vi "MMI_PEPS_StrDismantle.vi"(1 "LogEvent":refnum<vi>, 2 "VCI_CAN_OBJ_R":T1) -> (0 "MMI_PEPS_CmdCluster":T2 {"任意门开启锁车报警" items=["无请求", "禁止", "启用", "预留"]; "天窗/遮阳帘关闭设置" items=["无请求", "天窗关闭", "遮阳帘关闭", "预留"]; "车窗透气开启设置" items=["无请求", "禁止", "启用", "预留"]; "前雨刮激活后雨刮" items=["无请求", "不激活", "激活", "预留"]; "AVM道路中标定请求" items=["无请求", "开始标定", "预留"]; "自动开关窗设置" items=["无请求", "RKE长按控制", "车钥匙控制", "预留"]; "迎宾灯功能开关" items=["无请求", "禁止", "启用", "预留"]; "钥匙忘车内锁车报警" items=["无请求", "禁止", "启用", "预留"]; "AVAS禁用设置" items=["无请求", "禁止", "启用", "预留"]; "电源非OFF锁车报警" items=["无请求", "禁止", "启用", "预留"]; "外后视镜倒车倾斜" items=["无请求", "禁止所有倾斜", "启用驾驶侧", "启用乘客侧", "启用所有侧"]})   [LabVIEW 2013]
uses:
  Log.ctl
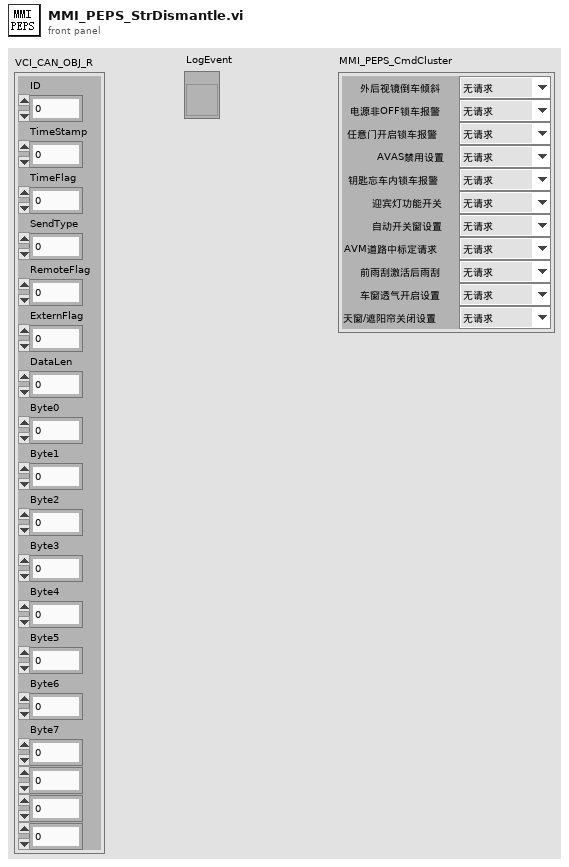
[diagram p1: front panel]
types:
  T1 = cluster{"ID":u32, "TimeStamp":u32, "TimeFlag":u8, "SendType":u8, "RemoteFlag":u8, "ExternFlag":u8, "DataLen":u8, "Byte0":u8, "Byte1":u8, "Byte2":u8, "Byte3":u8, "Byte4":u8, "Byte5":u8, "Byte6":u8, "Byte7":u8, u8, u8, u8}
  T2 = cluster{"外后视镜倒车倾斜":u16, "电源非OFF锁车报警":u16, " 任意门开启锁车报警":u16, "AVAS禁用设置":u16, "钥匙忘车内锁车报警":u16, "迎宾灯功能开关":u16, "自动开关窗设置":u16, "AVM道路中标定请求":u16, "前雨刮激活后雨刮":u16, "车窗透气开启设置":u16, "天窗/遮阳帘关闭设置":u16}
  T3 = typedef "Log.ctl" = cluster{"Event":string, "Value":variant}
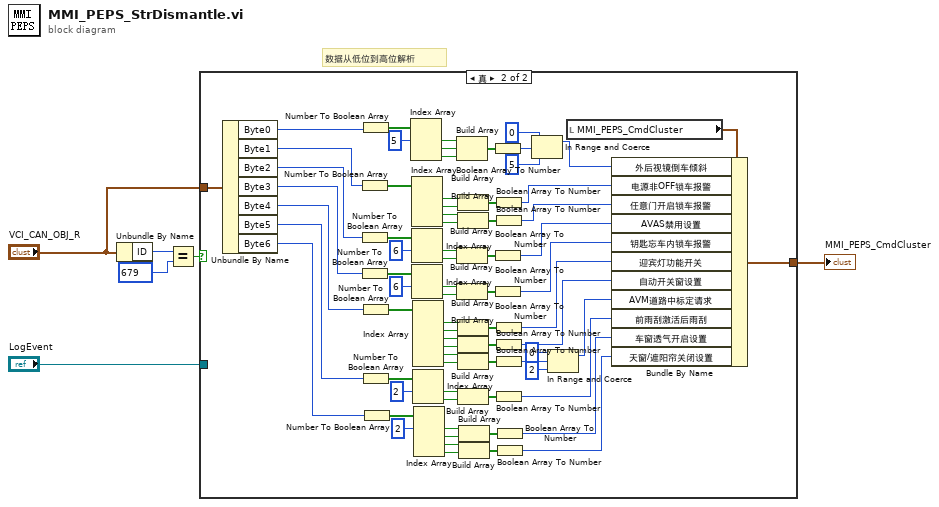
[diagram p0: block diagram]
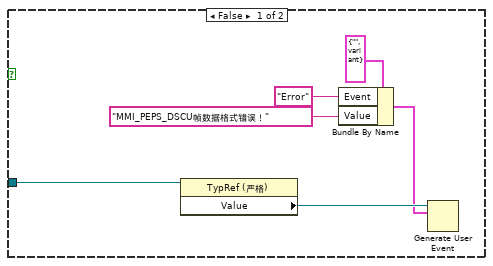
[diagram p2: hidden frame]
diagram:
  # "数据从低位到高位解析"
  n1 = Unbundle By Name("VCI_CAN_OBJ_R") -> ("ID"=w5:u32)
  n2 = Equal?(x=w5, y=u16 679) -> (x = y?=w3:bool)
  n3 = case shown="真" w3 {
    tunnel: [_ w21] -> w6
    tunnel: "VCI_CAN_OBJ_R" -> [_ w20]
    tunnel: "LogEvent" -> [w8 _]
    frame False {
      n4 = property class="TypRef (严格)"(reference=w8) -> ("Value"=w12:refnum<user-event>)  [unwired: 1 in, 2 out]
      n5 = Bundle By Name(cluster=T3 {"Event"="", "Value"=variant} ("Log"), "Event"="Error", "Value"="MMI_PEPS_DSCU帧数据格式错误！" ("消息")) -> (w9:T3)
      n6 = Generate User Event(user event=w12, event data cluster=w9) -> ()  [unwired: 2 in, 2 out]
    }
    frame True {
      n7 = Unbundle By Name(w20) -> ("Byte0"=w19:u8, "Byte1"=w18:u8, "Byte2"=w17:u8, "Byte3"=w16:u8, "Byte4"=w15:u8, "Byte5"=w14:u8, "Byte6"=w13:u8)
      n8 = Number To Boolean Array(number=w18) -> (Boolean array=w74:bool[])
      n9 = Number To Boolean Array(number=w17) -> (Boolean array=w65:bool[])
      n10 = Number To Boolean Array(number=w16) -> (Boolean array=w55:bool[])
      n11 = Number To Boolean Array(number=w19) -> (Boolean array=w84:bool[])
      n12 = Number To Boolean Array(number=w15) -> (Boolean array=w53:bool[])
      n13 = Number To Boolean Array(number=w14) -> (Boolean array=w37:bool[])
      n14 = Number To Boolean Array(number=w13) -> (Boolean array=w27:bool[])
      n15 = Index Array(array=w84, index #1=5 ("索引")) -> (element #1=w82:bool, element #2=w81:bool, element #3=w80:bool)  [unwired: 2 in]
      n16 = Index Array(array=w74) -> (element #1=w73:bool, element #2=w72:bool, element #3=w69:bool, element #4=w68:bool)  [unwired: 4 in]
      n17 = Index Array(array=w65, index #1=6 ("索引")) -> (element #1=w62:bool, element #2=w61:bool)  [unwired: 1 in]
      n18 = Index Array(array=w55, index #1=6 ("索引")) -> (element #1=w58:bool, element #2=w59:bool)  [unwired: 1 in]
      n19 = Index Array(array=w53) -> (element #1=w51:bool, element #2=w50:bool, element #3=w47:bool, element #4=w46:bool, element #5=w43:bool, element #6=w42:bool)  [unwired: 6 in]
      n20 = Index Array(array=w37, index #1=2 ("索引")) -> (element #1=w33:bool, element #2=w34:bool)  [unwired: 1 in]
      n21 = Index Array(array=w27, index #1=2 ("索引")) -> (element #1=w31:bool, element #2=w30:bool, element #3=w24:bool, element #4=w23:bool)  [unwired: 3 in]
      n22 = Build Array(w82, w81, w80) -> (w79:bool[])
      n23 = Build Array(w62, w61) -> (w63:bool[])
      n24 = Build Array(w58, w59) -> (w57:bool[])
      n25 = Build Array(w73, w72) -> (w71:bool[])
      n26 = Build Array(w69, w68) -> (w67:bool[])
      n27 = Build Array(w51, w50) -> (w52:bool[])
      n28 = Build Array(w47, w46) -> (w48:bool[])
      n29 = Build Array(w43, w42) -> (w44:bool[])
      n30 = Build Array(w33, w34) -> (w35:bool[])
      n31 = Build Array(w31, w30) -> (w29:bool[])
      n32 = Build Array(w24, w23) -> (w25:bool[])
      n33 = Boolean Array To Number(Boolean array=w79) -> (number=w78:u32)
      n34 = Boolean Array To Number(Boolean array=w63) -> (number=w60:u32)
      n35 = Boolean Array To Number(Boolean array=w57) -> (number=w54:u32)
      n36 = Boolean Array To Number(Boolean array=w71) -> (number=w70:u32)
      n37 = Boolean Array To Number(Boolean array=w67) -> (number=w66:u32)
      n38 = Boolean Array To Number(Boolean array=w52) -> (number=w49:u32)
      n39 = Boolean Array To Number(Boolean array=w48) -> (number=w45:u32)
      n40 = Boolean Array To Number(Boolean array=w44) -> (number=w41:u32)
      n41 = Boolean Array To Number(Boolean array=w35) -> (number=w32:u32)
      n42 = Boolean Array To Number(Boolean array=w29) -> (number=w26:u32)
      n43 = Boolean Array To Number(Boolean array=w25) -> (number=w22:u32)
      n44 = In Range and Coerce(upper limit=u32 0 ("上限"), x=w78, lower limit=u32 5 ("下限")) -> (coerced(x)=w77:u32)  [unwired: 1 out]
      n45 = In Range and Coerce(upper limit=u32 0 ("上限"), x=w41, lower limit=u32 2 ("下限")) -> (coerced(x)=w38:u32)  [unwired: 1 out]
      n46 = local read "MMI_PEPS_CmdCluster"() -> (w85:T2)
      n47 = Bundle By Name(cluster=w85, "外后视镜倒车倾斜"=w77, "电源非OFF锁车报警"=w70, "任意门开启锁车报警"=w66, "AVAS禁用设置"=w60, "钥匙忘车内锁车报警"=w54, "迎宾灯功能开关"=w49, "自动开关窗设置"=w45, "AVM道路中标定请求"=w38, "前雨刮激活后雨刮"=w32, "车窗透气开启设置"=w26, "天窗/遮阳帘关闭设置"=w22) -> (w21:T2)
    }
  }
  "MMI_PEPS_CmdCluster" <- w6
